vi "初级生产力线程.vi"() -> (3 "data":T1)   [LabVIEW 2016, in "main.lvlib"]
uses:
  main.lvlib
  Primary Productivity/Primary Productivity.lvclass
  <vilib>/ptbypt/NI_PtbyPt.lvlib
panel:
  in  "停止":bool
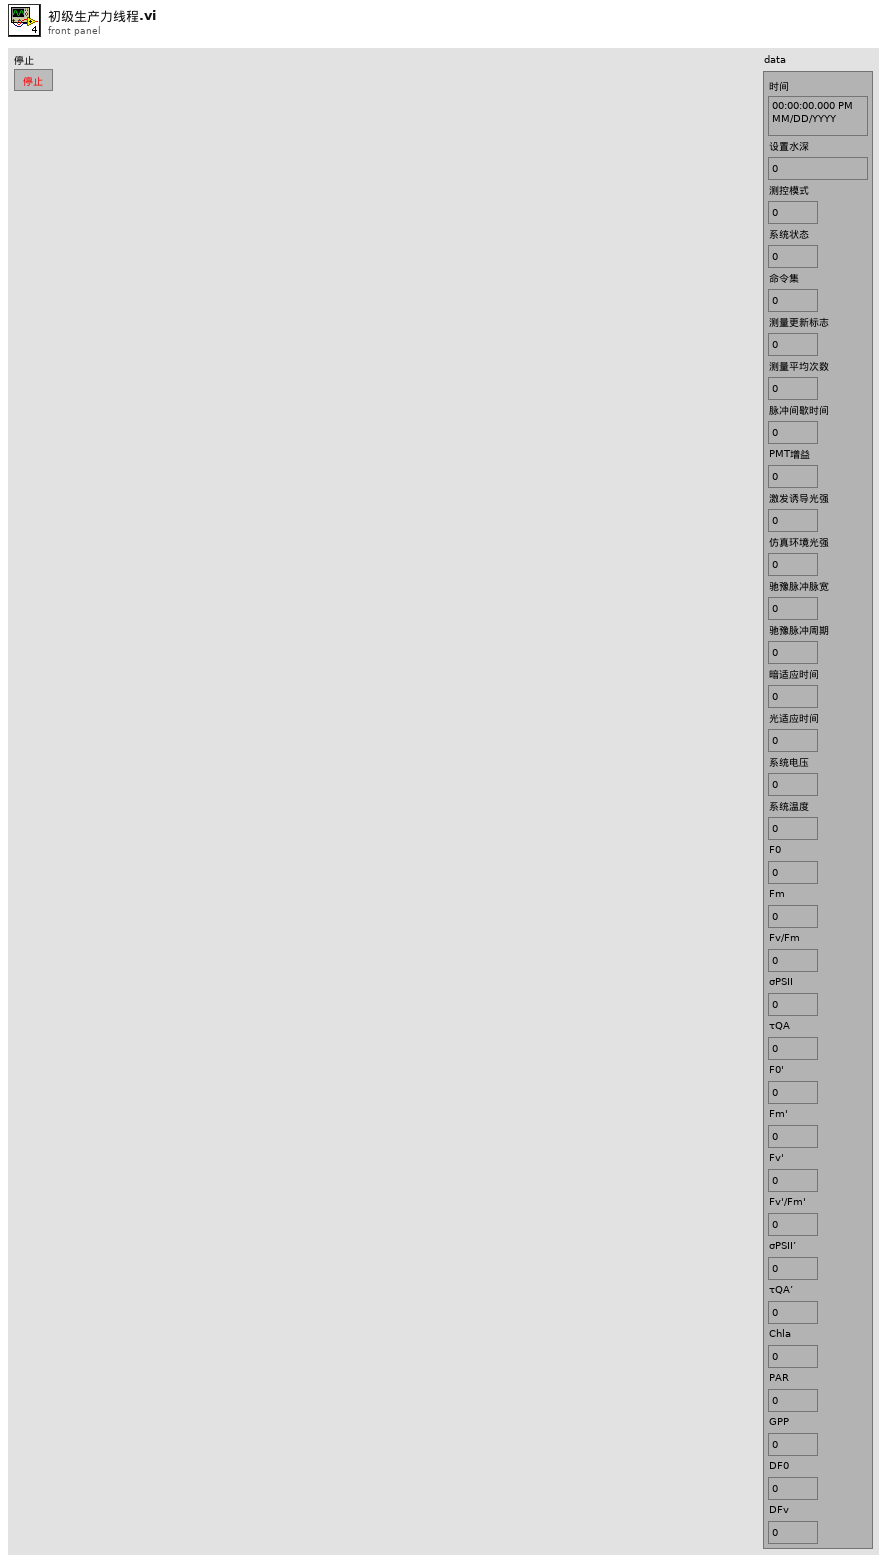
[diagram p1: front panel]
types:
  T1 = cluster{"时间":timestamp, "设置水深":sgl, "测控模式":u16, "系统状态":u16, "命令集":u16, "测量更新标志":u16, "测量平均次数":u16, "脉冲间歇时间":u16, "PMT增益":u16, "激发诱导光强":u16, "仿真环境光强":u16, "驰豫脉冲脉宽":u16, "驰豫脉冲周期":u16, "暗适应时间":u16, "光适应时间":u16, "系统电压":sgl, "系统温度":sgl, "F0":sgl, "Fm":sgl, "Fv/Fm":sgl, "σPSII":sgl, "τQA":sgl, "F0'":sgl, "Fm'":sgl, "Fv'":sgl, "Fv'/Fm'":sgl, "σPSII’":sgl, "τQA’":sgl, "Chla":sgl, "PAR":sgl, "GPP":sgl, "DF0":sgl, "DFv":sgl}
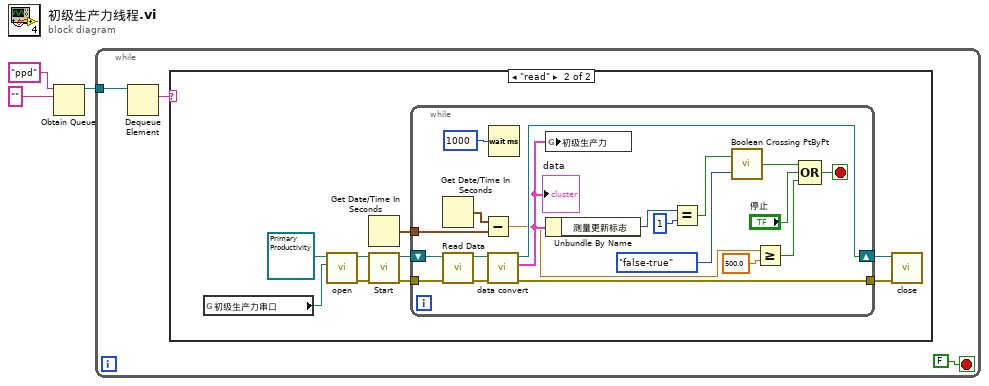
[diagram p0: block diagram]
diagram:
  n1 = Obtain Queue(name (unnamed)="ppd" ("名称（未命名）"), element data type="") -> (queue out=w1:refnum<queue>)  [unwired: 3 in, 2 out]
  n2 = while {
    tunnel: w1 -> [w6]
    stop <- FALSE stop-if-true
    n3 = Dequeue Element(queue=w6) -> (element=w5:string)  [unwired: 2 in, 3 out]
    n4 = case shown="\"read\"" w5 {
      frame "假", Default {
      }
      frame "read" {
        n5 = global read "全局断电保存变量.vi" "初级生产力串口"() -> (w8:refnum<visa-resource-name>)
        n6 = call "open.vi"("VISA resource name"=w8, "Primary Productivity 输入"=refnum<class "Primary Productivity.lvclass"> refnum ("Primary Productivity.lvclass")) -> ("error out"=w11:errorcluster, "Primary Productivity 输出"=w10:refnum<class "Primary Productivity.lvclass">)  [unwired: 8 in]
        n7 = Get Date/Time In Seconds() -> (seconds since 1Jan1904=w7:timestamp)
        n8 = call "Start.vi"("error in (no error)"=w11, "Primary Productivity 输入"=w10) -> ("error out"=w13:errorcluster, "Primary Productivity 输出"=w12:refnum<class "Primary Productivity.lvclass">)  [unwired: 8 in]
        n9 = while {
          shift-right: [w31] -> w14
          shift-left: w12 -> [w35]
          tunnel: w13 -> [w34]
          tunnel: [w29] -> w15
          tunnel: w7 -> [w19]
          stop <- w26 stop-if-true
          n10 = Get Date/Time In Seconds() -> (seconds since 1Jan1904=w20:timestamp)
          n11 = call "Read Data.vi"("error in (no error)"=w34, "Primary Productivity 输入"=w35) -> ("error out"=w32:errorcluster, "Primary Productivity 输出"=w33:refnum<class "Primary Productivity.lvclass">)  [unwired: 8 in]
          n12 = Subtract(x=w20, y=w19) -> (x-y=w18:dbl)
          n13 = call "data convert.vi"("error in (no error)"=w32, "Primary Productivity 输入"=w33) -> ("error out"=w29:errorcluster, "data"=w22:T1, "Primary Productivity 输出"=w31:refnum<class "Primary Productivity.lvclass">)  [unwired: 7 in]
          "data" <- w22
          n14 = Wait (ms)(milliseconds to wait=u32 1000 ("等待时间（毫秒）")) -> ()  [unwired: 1 out]
          n15 = global write "全局非断电保持变量.vi" "初级生产力"(w22) -> ()
          n16 = Unbundle By Name(w22) -> ("测量更新标志"=w28:u16)
          n17 = Equal?(x=w28, y=u16 1) -> (x = y?=w25:bool)
          n18 = call <vilib>:"Boolean Crossing PtByPt.vi"("direction"=enum16{"either", "false-true", "true-false"}."false-true", "input"=w25) -> ("crossing"=w23:bool)  [unwired: 1 in]
          n19 = Greater Or Equal?(x=w18, y=500.0) -> (x >= y?=w16:bool)
          n20 = Compound Arithmetic op=OR ("复合运算")(w23, "停止", w16) -> (w26:bool)
        }
        n21 = call "close.vi"("error in (no error)"=w15, "Primary Productivity 输入"=w14) -> ()  [unwired: 8 in, 2 out]
      }
    }
  }
